vi "校准中 (子VI).vi"(0 "曲线模型":refnum<vi>, 1 "校准按钮":refnum<vi>) -> ()   [LabVIEW 2016, in "斯坦道氨氮.lvlib"]
uses:
  <vilib>/ptbypt/NI_PtbyPt.lvlib
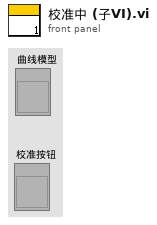
[diagram p1: front panel]
types:
  T1 = enum8{"Enabled", "Disabled", "Disabled and Grayed Out"}
  T2 = cluster{"系统时间":timestamp, "工作状态":enum16{"空闲", "水样测试", "标样核查", "零点核查", "跨度核查", "空白测试", "平行样测试", "加标回收", "空白校准", "标样校准", "初始化（清洗）"}, "测量模式":enum16{"待机", "连续模式", "周期模式", "定点模式", "受控模式", "手动模式"}, "告警代码":u16, "故障代码":u16, "日志代码":u16, "软件版本":u16, "F0":sgl, "F1":sgl, "F2":sgl, "F3":sgl, "T":sgl, "H":sgl, "id":u16, "flowid":u16, "量程":u16, "总磷控温温度1":sgl, "营养盐控温温度2":sgl, "ADC":sgl}
  T3 = enum16{"空闲", "水样测试", "标样核查", "零点核查", "跨度核查", "空白测试", "平行样测试", "加标回收", "空白校准", "标样校准", "初始化（清洗）"}
  T4 = cluster{"因子编码":u32, "单位":u16, "标样参考值":sgl, "水样数据时间":timestamp, "水样实测值":sgl, "水样数据标识":string, "标样数据时间":timestamp, "标样实测值":sgl, "标样数据标识":string, "空白数据时间":timestamp, "空白实测值":sgl, "空白数据标识":string, "零点核查数据时间":timestamp, "零点核查实测值":sgl, "零点核查数据标识":string, "跨度核查数据时间":timestamp, "跨度核查实测值":sgl, "跨度核查数据标识":string, "加标回收数据时间":timestamp, "加标回收实测值":sgl, "加标回收数据标识":string, "平行样数据时间":timestamp, "平行样实测值":sgl, "平行样数据标识":string, "F0":sgl, "F1":sgl, "F2":sgl, "F3":sgl, "F4":sgl, "F5":sgl, "F6":sgl, "F7":sgl, "温度":sgl, "湿度":sgl, "X值":sgl, "fidrange":u16}
  T5 = cluster{"Value":dbl, "Value 2":dbl, "Value 3":dbl, "Value 4":dbl, "Value 5":dbl}
  T6 = cluster{"测量量程":dbl, "测量精度":dbl, "测量间隔":dbl, "消解温度":dbl, "消解时长":dbl, "空白校准时间":timestamp, "曲线截距":dbl, "曲线斜率":dbl, "测量检出限":dbl, "测量信号值":dbl, "线性相关系数":dbl, "二次多项式系数":dbl, "标样校准时间":timestamp, "单位":u16}
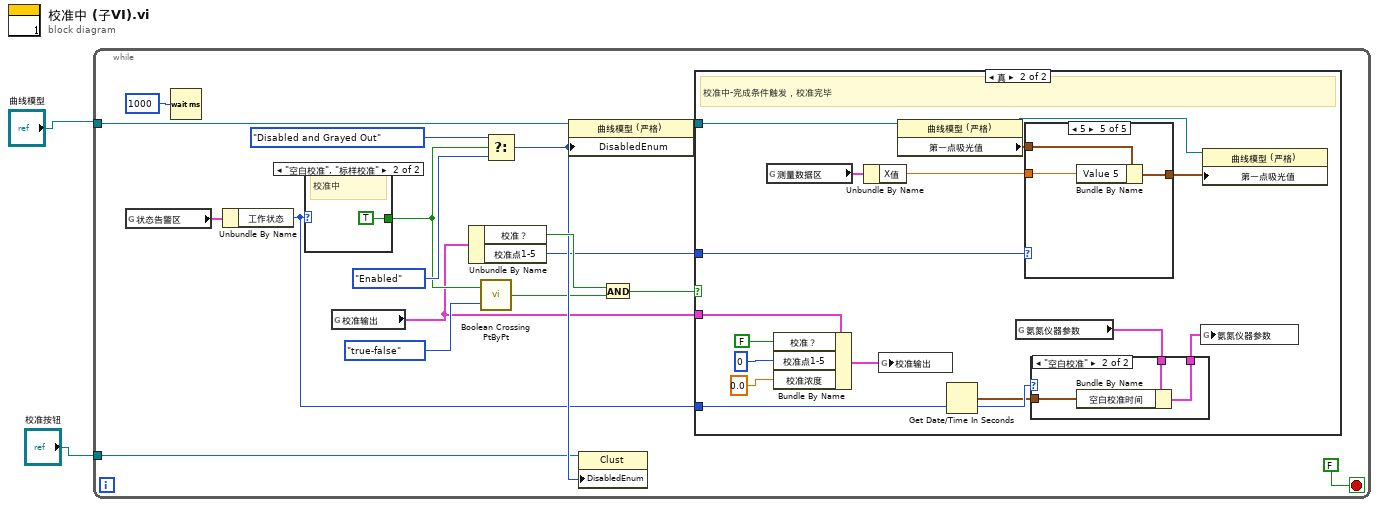
[diagram p0: block diagram]
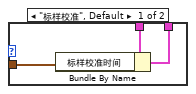
[diagram p3: hidden frame]
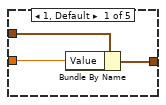
[diagram p4: hidden frame]
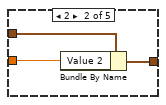
[diagram p5: hidden frame]
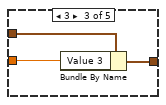
[diagram p6: hidden frame]
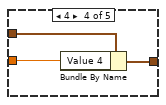
[diagram p7: hidden frame]
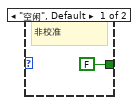
[diagram p8: hidden frame]
diagram:
  n1 = while {
    tunnel: "校准按钮" -> [w6]
    tunnel: "曲线模型" -> [w5]
    stop <- FALSE stop-if-true
    n2 = global read "VAR氨氮全局变量.vi" "状态告警区"() -> (w19:T2)
    n3 = Wait (ms)(milliseconds to wait=u32 1000 ("等待时间（毫秒）")) -> ()  [unwired: 1 out]
    n4 = Unbundle By Name(w19) -> ("工作状态"=w3:T3)
    n5 = case shown="\"空白校准\", \"标样校准\"" w3 {
      tunnel: [FALSE TRUE] -> w9
      frame "空闲", Default {
        # "非校准"
      }
      frame "空白校准", "标样校准" {
        # "校准中"
      }
    }
    n6 = global read "氨氮断电保存全局变量.vi" "校准输出"() -> (w4:cluster{"校准？":bool, "校准点1-5":u16, "校准浓度":dbl})
    n7 = Unbundle By Name(w4) -> ("校准？"=w18:bool, "校准点1-5"=w10:u16)
    n8 = call <vilib>:"Boolean Crossing PtByPt.vi"("direction"=enum16{"either", "false-true", "true-false"}."true-false", "input"=w9) -> ("crossing"=w7:bool)  [unwired: 1 in]
    n9 = Select(t=T1."Disabled and Grayed Out" ("禁用"), s=w9, f=T1."Enabled" ("禁用")) -> (s? t:f=w13:T1)
    n10 = property class="曲线模型 (严格)"(reference=w5, "DisabledEnum"=w13) -> (reference out=w11:refnum<vi>)  [unwired: 1 in, 1 out]
    n11 = property class="Clust"(reference=w6, "DisabledEnum"=w13) -> ()  [unwired: 1 in, 2 out]
    n12 = And(x=w18, y=w7) -> (x .and. y?=w12:bool)
    n13 = case shown="真" w12 {
      tunnel: w11 -> [_ w35]
      tunnel: w10 -> [_ w33]
      tunnel: w4 -> [_ w30]
      tunnel: w3 -> [_ w23]
      frame False {
      }
      frame True {
        # "校准中-完成条件触发，校准完毕"
        n14 = global read "VAR氨氮全局变量.vi" "测量数据区"() -> (w25:T4)
        n15 = Bundle By Name(cluster=w30, "校准？"=FALSE ("校准.校准？"), "校准点1-5"=u16 0 ("校准.校准点1-5"), "校准浓度"=0.0 ("校准.校准浓度")) -> (w26:cluster{"校准？":bool, "校准点1-5":u16, "校准浓度":dbl})
        n16 = Unbundle By Name(w25) -> ("X值"=w24:sgl)
        n17 = global write "氨氮断电保存全局变量.vi" "校准输出"(w26) -> ()
        n18 = property class="曲线模型 (严格)"(reference=w35) -> (reference out=w34:refnum<vi>, "第一点吸光值"=w32:T5)  [unwired: 1 in, 1 out]
        n19 = Get Date/Time In Seconds() -> (seconds since 1Jan1904=w20:timestamp)
        n20 = global read "氨氮断电保存全局变量.vi" "氨氮仪器参数"() -> (w22:T6)
        n21 = case shown="5" w33 {
          tunnel: w32 -> [w44 w47 w50 w53 w55]
          tunnel: [w43 w46 w49 w52 w56] -> w31
          tunnel: w24 -> [w42 w45 w48 w51 w54]
          frame 1, Default {
            n22 = Bundle By Name(cluster=w44, "Value"=w42) -> (w43:T5)
          }
          frame 2 {
            n23 = Bundle By Name(cluster=w47, "Value 2"=w45) -> (w46:T5)
          }
          frame 3 {
            n24 = Bundle By Name(cluster=w50, "Value 3"=w48) -> (w49:T5)
          }
          frame 4 {
            n25 = Bundle By Name(cluster=w53, "Value 4"=w51) -> (w52:T5)
          }
          frame 5 {
            n26 = Bundle By Name(cluster=w55, "Value 5"=w54) -> (w56:T5)
          }
        }
        n27 = case shown="\"空白校准\"" w23 {
          tunnel: w22 -> [w38 w40]
          tunnel: [w37 w39] -> w21
          tunnel: w20 -> [w36 w41]
          frame "标样校准", Default {
            n28 = Bundle By Name(cluster=w38, "标样校准时间"=w36) -> (w37:T6)
          }
          frame "空白校准" {
            n29 = Bundle By Name(cluster=w40, "空白校准时间"=w41) -> (w39:T6)
          }
        }
        n30 = global write "氨氮断电保存全局变量.vi" "氨氮仪器参数"(w21) -> ()
        n31 = property class="曲线模型 (严格)"(reference=w34, "第一点吸光值"=w31) -> ()  [unwired: 1 in, 2 out]
      }
    }
  }
